vi "Write String Data.vi"(8 "error in (no error)":errorcluster, 10 "String Data":string, 11 "class string in":refnum<class "Parent.lvclass">) -> (0 "error out":errorcluster, 3 "class string out":refnum<class "Parent.lvclass">)   [LabVIEW 2023, in "Parent.lvclass"]
doc: "This is a member VI of Parent.lvclass, which sets the string data for Parent.ctl, a data member of Parent.lvclass."
uses:
  Parent.lvclass
  Parent.lvclass/Parent.ctl
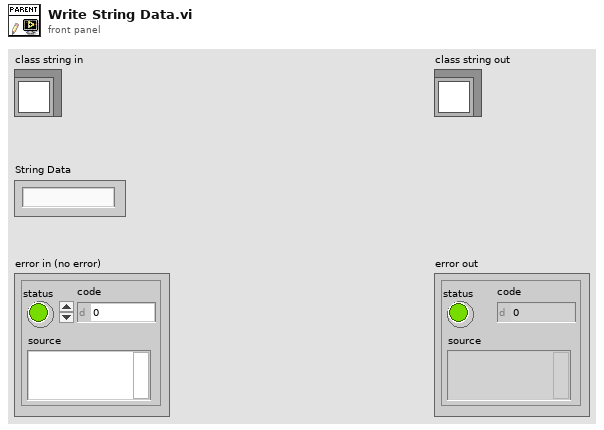
[diagram p1: front panel]
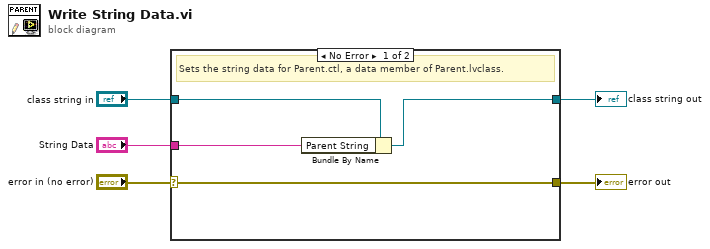
[diagram p0: block diagram]
diagram:
  n1 = case shown="No Error" "error in (no error)" {
    selector: "error in (no error)" -> [w9 w10]
    tunnel: [w9 w10] -> w4
    tunnel: [w7 w11] -> w2
    tunnel: "class string in" -> [w8 w11]
    tunnel: "String Data" -> [w6 _]
    frame No Error {
      # "Sets the string data for Parent.ctl, a data member of Parent.lvclass."
      n2 = Bundle By Name(cluster=w8, "Parent String"=w6) -> (w7:refnum<class "Parent.lvclass">)
    }
    frame Error {
    }
  }
  "error out" <- w4
  "class string out" <- w2
